vi "Frame Pass.vi"(11 "Color Box":u32(colorbox)=6618880) -> (3 "Frames":T1[](array[typedef]))   [LabVIEW 2019, in "LED Matrix Host.lvlib"]
uses:
  LED Matrix Host.lvlib
  Public/Controls/Frame.ctl
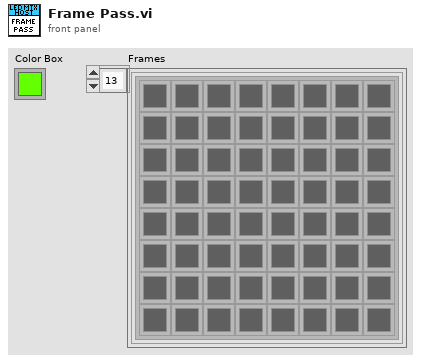
[diagram p1: front panel]
types:
  T1 = typedef "LED Matrix Host.lvlib/Frame.ctl" = cluster{"Matrix":u32[][]}
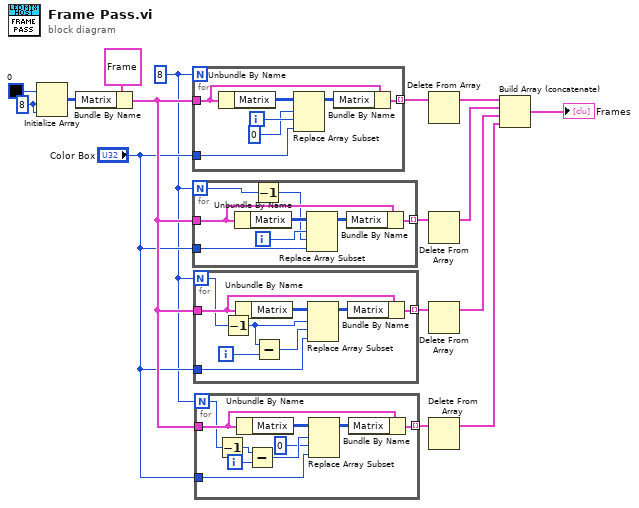
[diagram p0: block diagram]
diagram:
  w9 = 8
  w13 = 8 ("dimension size")
  n1 = Initialize Array(u32 0 ("Color Box"), w13, w13) -> (w14:u32[][])
  n2 = Bundle By Name(cluster=T1 {"Matrix"=[[0, 0, 0, 0, 0, 0, 0, 0], [16777222, 16777222, 0, 0, 0, 0, 0, 0], [0, 0, 0, 0, 0, 0, 0, 0], [0, 0, 0, 0, 0, 0, 0, 0], [0, 0, 0, 0, 0, 0, 0, 0], [0, 0, 0, 0, 0, 0, 0, 0], [0, 0, 0, 0, 0, 0, 0, 0], [16777222, 0, 0, 0, 0, 0, 0, 16777222]]} ("Matrix"), "Matrix"=w14) -> (w11:T1)
  n3 = for {
    N: w9 -> [_]
    tunnel: w11 -> [w23]
    tunnel: "Color Box" -> [w18]
    tunnel: [w22] -> w8 mode=indexing
    i -> [w21]
    n4 = Unbundle By Name(w23) -> ("Matrix"=w20:u32[][])
    n5 = Replace Array Subset(array=w20, new element=w18, index (row)=0 ("disabled index (row)"), index (col)=w21) -> (w19:u32[][])
    n6 = Bundle By Name(cluster=w23, "Matrix"=w19) -> (w22:T1)
  }
  n7 = for {
    N: w9 -> [w25]
    tunnel: w11 -> [w31]
    tunnel: "Color Box" -> [w27]
    tunnel: [w30] -> w6 mode=indexing
    i -> [w26]
    n8 = Unbundle By Name(w31) -> ("Matrix"=w29:u32[][])
    n9 = Decrement(x=w25) -> (x-1=w24:i32)
    n10 = Replace Array Subset(array=w29, new element=w27, index (row)=w26, index (col)=w24) -> (w28:u32[][])
    n11 = Bundle By Name(cluster=w31, "Matrix"=w28) -> (w30:T1)
  }
  n12 = for {
    N: w9 -> [w33]
    tunnel: w11 -> [w40]
    tunnel: "Color Box" -> [w36]
    tunnel: [w39] -> w4 mode=indexing
    i -> [w35]
    n13 = Decrement(x=w33) -> (x-1=w32:i32)
    n14 = Unbundle By Name(w40) -> ("Matrix"=w38:u32[][])
    n15 = Subtract(x=w32, y=w35) -> (x-y=w34:i32)
    n16 = Replace Array Subset(array=w38, new element=w36, index (row)=w32, index (col)=w34) -> (w37:u32[][])
    n17 = Bundle By Name(cluster=w40, "Matrix"=w37) -> (w39:T1)
  }
  n18 = for {
    N: w9 -> [w42]
    tunnel: w11 -> [w50]
    tunnel: "Color Box" -> [w46]
    tunnel: [w49] -> w2 mode=indexing
    i -> [w45]
    n19 = Decrement(x=w42) -> (x-1=w41:i32)
    n20 = Unbundle By Name(w50) -> ("Matrix"=w48:u32[][])
    n21 = Subtract(x=w41, y=w45) -> (x-y=w44:i32)
    n22 = Replace Array Subset(array=w48, new element=w46, index (row)=w44, index (col)=0 ("disabled index (col)")) -> (w47:u32[][])
    n23 = Bundle By Name(cluster=w50, "Matrix"=w47) -> (w49:T1)
  }
  n24 = Delete From Array(array=w8) -> (array with subset deleted=w7:T1[])  [unwired: 2 in, 1 out]
  n25 = Delete From Array(array=w6) -> (array with subset deleted=w5:T1[])  [unwired: 2 in, 1 out]
  n26 = Delete From Array(array=w4) -> (array with subset deleted=w3:T1[])  [unwired: 2 in, 1 out]
  n27 = Delete From Array(array=w2) -> (array with subset deleted=w1:T1[])  [unwired: 2 in, 1 out]
  n28 = Build Array (concatenate)(w7, w5, w3, w1) -> (→"Frames":T1[])
